vi "evaluateVonKarman.vi"(8 "a":dbl format="%#_4g", 9 "frequencies":dbl[](array[numeric]), 10 "lambda":dbl, 11 "vonKarmanFitEquation":string) -> (3 "Cluster":cluster{"frequencies":dbl[], "Y Values":dbl[]})   [LabVIEW 2018]
uses:
  <vilib>/gmath/NI_Gmath.lvlib
panel:
  out "result string":string
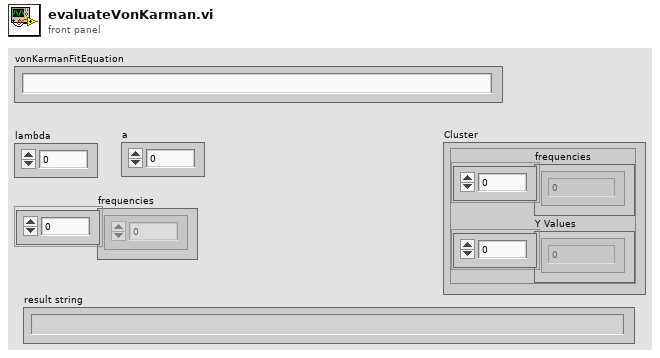
[diagram p1: front panel]
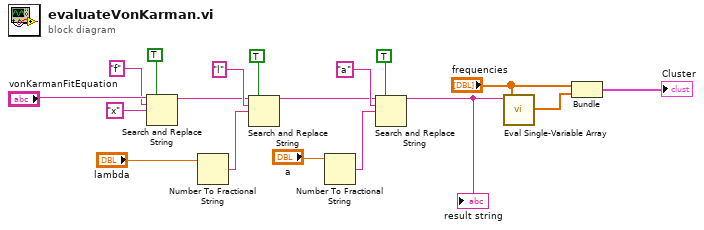
[diagram p0: block diagram]
diagram:
  n1 = Search and Replace String(replace all?=TRUE ("replace all? (F)"), input string="vonKarmanFitEquation", search string="f", replace string="x" ("replace string (\"\")")) -> (result string=w9:string)  [unwired: 4 in, 3 out]
  n2 = Number To Fractional String(number="lambda") -> (F-format string=w8:string)  [unwired: 3 in]
  n3 = Search and Replace String(replace all?=TRUE ("replace all? (F)"), input string=w9, search string="l", replace string=w8) -> (result string=w3:string)  [unwired: 4 in, 3 out]
  n4 = Number To Fractional String(number="a") -> (F-format string=w7:string)  [unwired: 3 in]
  n5 = Search and Replace String(replace all?=TRUE ("replace all? (F)"), input string=w3, search string="a", replace string=w7) -> (result string=w4:string)  [unwired: 4 in, 3 out]
  "result string" <- w4
  n6 = call <vilib>:"Eval Single-Variable Array.vi"("X Values"="frequencies", "formula"=w4) -> ("Y Values"=w16:dbl[])  [unwired: 1 in, 1 out]
  n7 = Bundle("frequencies"="frequencies", "Y Values"=w16) -> (→"Cluster":cluster{"frequencies":dbl[], "Y Values":dbl[]})  [unwired: 1 in]
